vi "Setup_Authentication.vi"() -> (0 "file path":path)   [LabVIEW 2016]
uses:
  <vilib>/Utility/config.llb/Read Key (String).vi
  <vilib>/Platform/browser.llb/Open URL in Default Browser (string).vi
  <vilib>/Utility/config.llb/Write Key (Boolean).vi
  <vilib>/Utility/config.llb/Write Key (String).vi
  <vilib>/Utility/config.llb/NI_LVConfig.lvlib
panel:
  in  "error in (no error)":errorcluster
  out "error out":errorcluster
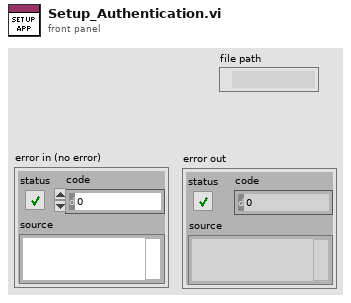
[diagram p1: front panel]
types:
  T1 = typedef "NI_LVConfig.lvlib/Config Data RefNum.ctl" = refnum<k1>
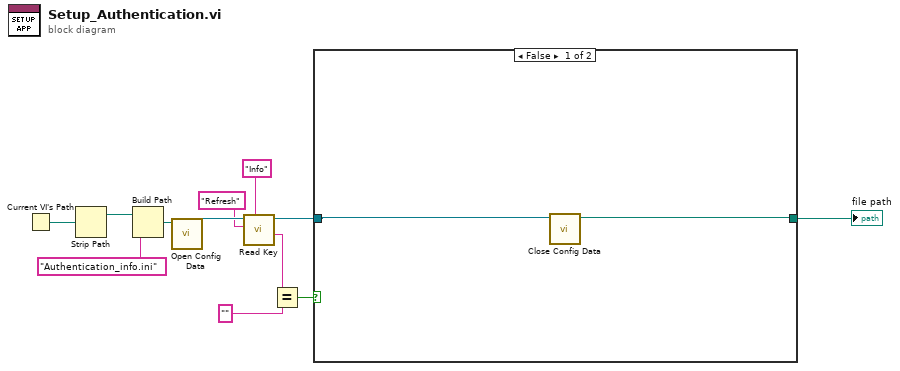
[diagram p0: block diagram]
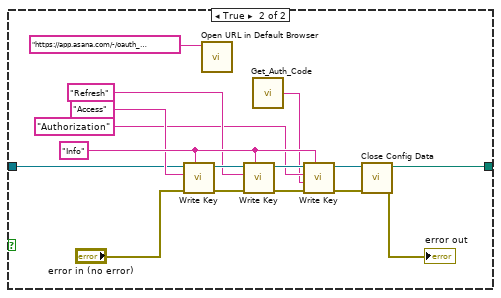
[diagram p2: hidden frame]
diagram:
  n1 = Current VI's Path() -> (path=w9:path)
  n2 = Strip Path(path=w9) -> (stripped path=w10:path)  [unwired: 1 out]
  n3 = Build Path(base path=w10, name or relative path="Authentication_info.ini") -> (appended path=w7:path)
  n4 = call <vilib>:"Open Config Data.vi"("configuration file path"=w7) -> ("refnum"=w11:T1)  [unwired: 8 in, 2 out]
  n5 = call-poly <vilib>:"Read Key.vi"("section"="Info", "key"="Refresh", "refnum"=w11) -> ("value"=w3:string, "refnum out"=w6:T1)  [unwired: 5 in, 2 out]
  n6 = Equal?(x=w3, y="") -> (x = y?=w2:bool)
  n7 = case shown="False" w2 {
    tunnel: w6 -> [w14 w17]
    tunnel: [w13 w15] -> w1
    frame False {
      n8 = call <vilib>:"Close Config Data.vi"("refnum"=w14) -> ("file path"=w13:path)  [unwired: 9 in, 1 out]
    }
    frame True {
      w25 = "Info"
      n9 = call-poly <vilib>:"Write Key.vi"("section"=w25, "error in (no error)"="error in (no error)", "key"="Access", "refnum"=w17) -> ("error out"=w29:errorcluster, "refnum out"=w28:T1)  [unwired: 5 in, 1 out]
      n10 = call-poly <vilib>:"Open URL in Default Browser.vi"("URL"="https://app.asana.com/-/oauth_authorize?response_type=code&client_id=1108428692000476&redirect_uri=https%3A%2F%2Fapp.asana.com%2Fapi%2F1.0&state=<STATE_PARAM>") -> ()  [unwired: 5 in, 2 out]
      n11 = call-poly <vilib>:"Write Key.vi"("section"=w25, "error in (no error)"=w29, "key"="Refresh", "refnum"=w28) -> ("error out"=w27:errorcluster, "refnum out"=w26:T1)  [unwired: 5 in, 1 out]
      n12 = call "Get_Auth_Code.vi"() -> ("Code Out"=w19:string)  [unwired: 1 in]
      n13 = call-poly <vilib>:"Write Key.vi"("section"=w25, "error in (no error)"=w27, "value"=w19, "key"="Authorization", "refnum"=w26) -> ("error out"=w23:errorcluster, "refnum out"=w24:T1)  [unwired: 4 in, 1 out]
      n14 = call <vilib>:"Close Config Data.vi"("error in (no error)"=w23, "refnum"=w24) -> ("error out"=→"error out":errorcluster, "file path"=w15:path)  [unwired: 8 in]
    }
  }
  "file path" <- w1
